vi "Min time calculation.vi"(8 "error in (no error)":errorcluster, 10 "Breakdown out Time Stamp":timestamp format="%<%.3X\n%Y-%m-%d>T", 11 "Breakdown inTime Stamp":timestamp format="%<%.3X\n%Y-%m-%d>T") -> (0 "error out":errorcluster, 2 "Time":string, 3 "min":dbl)   [LabVIEW 2017]
panel:
  # "2020-09-07 22:56:13"
  # "2020-09-08 0:06:51"
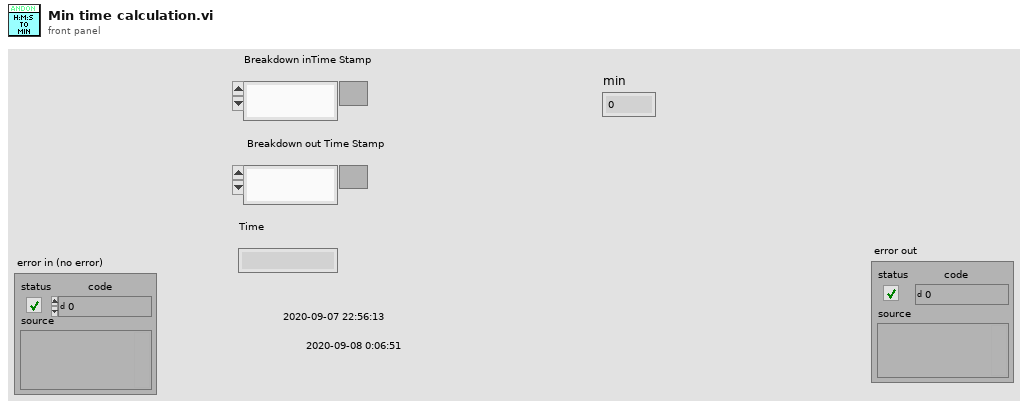
[diagram p1: front panel]
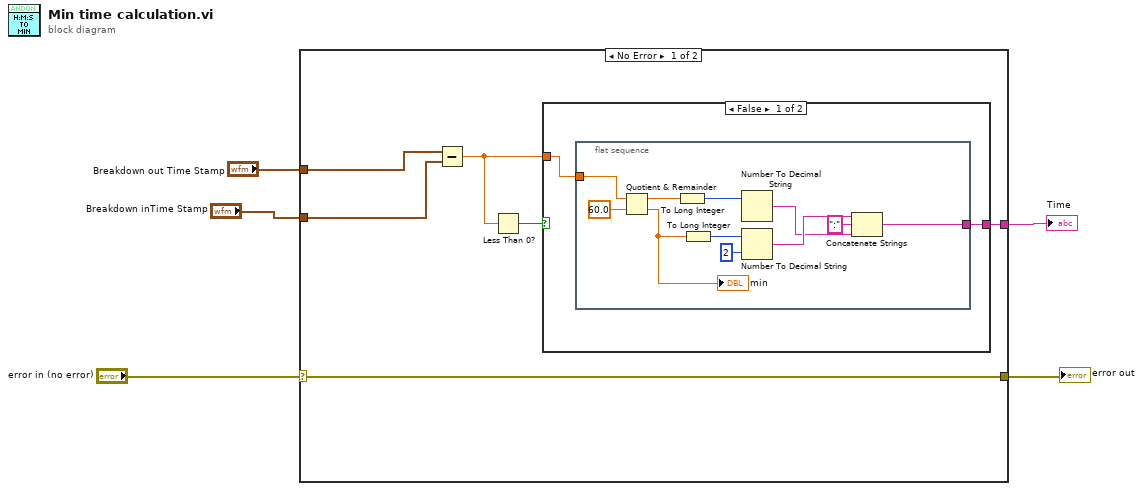
[diagram p0: block diagram]
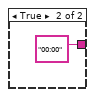
[diagram p2: hidden frame]
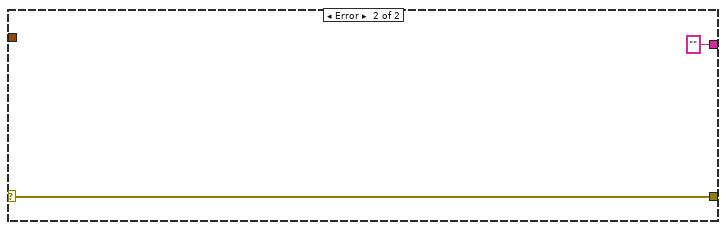
[diagram p3: hidden frame]
diagram:
  n1 = case shown="No Error" "error in (no error)" {
    selector: "error in (no error)" -> [w11 w27]
    tunnel: [w11 w27] -> w4
    tunnel: "Breakdown inTime Stamp" -> [w6 _]
    tunnel: "Breakdown out Time Stamp" -> [w7 _]
    tunnel: [w8 ""] -> w1
    frame No Error {
      n2 = Subtract(x=w7, y=w6) -> (x-y=w10:dbl)
      n3 = Less Than 0?(x=w10) -> (x < 0?=w9:bool)
      n4 = case shown="False" w9 {
        tunnel: w10 -> [w13 _]
        tunnel: [w12 "00:00"] -> w8
        frame False {
          n5 = flat-sequence {
            tunnel: [w18] -> w12
            tunnel: w13 -> [w20]
            frame #0 {
              n6 = Quotient & Remainder(x=w20, y=60.0) -> (x-y*floor(x/y)=w23:dbl, floor(x/y)=w19:dbl)
              "min" <- w19
              n7 = To Long Integer(number=w23) -> (32bit integer=w17:i32)
              n8 = To Long Integer(number=w19) -> (32bit integer=w21:i32)
              n9 = Number To Decimal String(number=w17) -> (decimal integer string=w14:string)  [unwired: 1 in]
              n10 = Number To Decimal String(number=w21, width (-)=i16 2) -> (decimal integer string=w15:string)
              n11 = Concatenate Strings(w15, ":" ("string"), w14) -> (w18:string)
            }
          }
        }
        frame True {
        }
      }
    }
    frame Error {
    }
  }
  "error out" <- w4
  "Time" <- w1
